vi "Mapping.vi"(4 "out_max":dbl, 5 "out_min":dbl, 9 "in_max":dbl, 10 "in_min":dbl, 11 "x":dbl) -> (2 "y":dbl)   [LabVIEW 2014]
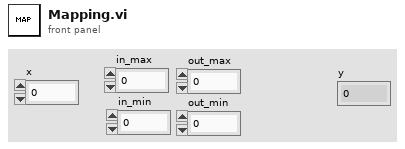
[diagram p1: front panel]
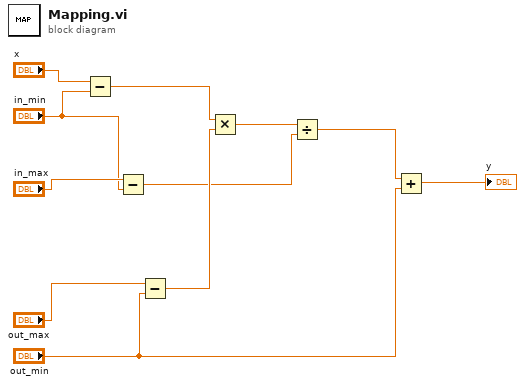
[diagram p0: block diagram]
diagram:
  n1 = Subtract(x="x", y="in_min") -> (x-y=w7:dbl)
  n2 = Subtract(x="in_max", y="in_min") -> (x-y=w4:dbl)
  n3 = Subtract(x="out_max", y="out_min") -> (x-y=w6:dbl)
  n4 = Multiply(x=w7, y=w6) -> (x*y=w5:dbl)
  n5 = Divide(x=w5, y=w4) -> (x/y=w3:dbl)
  n6 = Add(x=w3, y="out_min") -> (x+y=→"y":dbl)
